vi "sound and graphics.vi"() -> ()   [LabVIEW 2018]
panel:
  out "new picture":picture
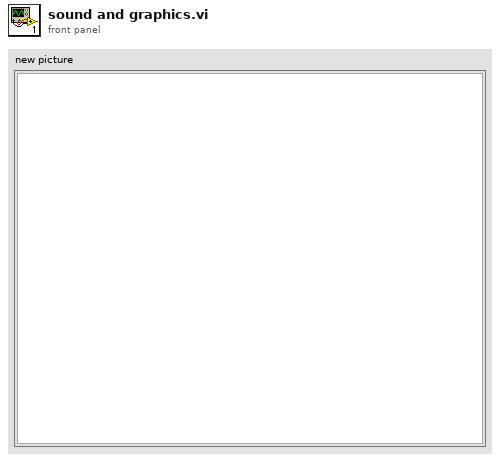
[diagram p1: front panel]
types:
  T1 = typedef "imagedata.ctl" = cluster{"image type":i32, "image depth":i32, "image":u8[], "mask":u8[], "colors":u32[], "Rectangle":cluster{"left":i16, "top":i16, "right":i16, "bottom":i16}}
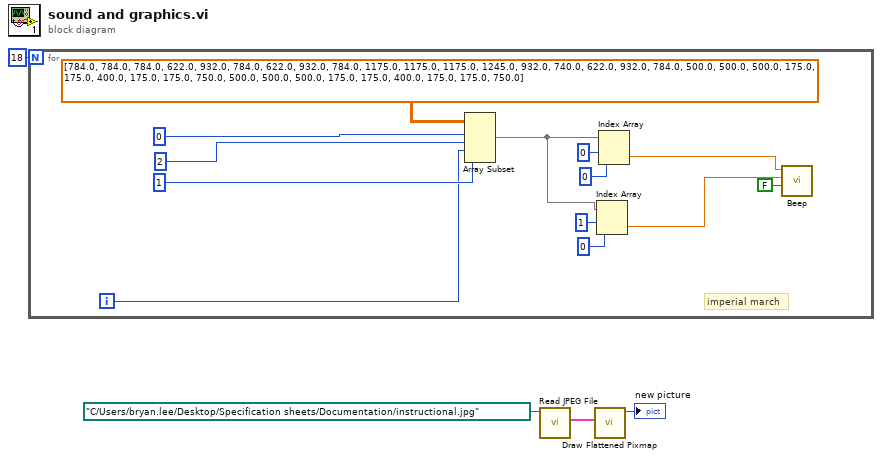
[diagram p0: block diagram]
diagram:
  n1 = for {
    N: 18 -> [_]
    i -> [w9]
    # "imperial march"
    n2 = Array Subset(array=dbl[][] [[784.0, 784.0, 784.0, 622.0, 932.0, 784.0, 622.0, 932.0, 784.0, 1175.0, 1175.0, 1175.0, 1245.0, 932.0, 740.0, 622.0, 932.0, 784.0], [500.0, 500.0, 500.0, 175.0, 175.0, 400.0, 175.0, 175.0, 750.0, 500.0, 500.0, 500.0, 175.0, 175.0, 400.0, 175.0, 175.0, 750.0]] ("Array"), index (row)=0 ("index"), length (row)=2 ("length"), index (col)=w9, length (col)=1 ("length")) -> (w10:dbl[][])
    n3 = Index Array(array=w10, index (row)=1, index (col)=0 ("disabled index (col)")) -> (element=w5:dbl)
    n4 = Index Array(array=w10, index (row)=0, index (col)=0 ("disabled index (col)")) -> (element=w6:dbl)
    n5 = call <vilib>:"Beep.vi"("use system alert? (T)"=FALSE, "duration (msec)"=w5, "frequency (Hz)"=w6) -> ()  [unwired: 9 in]
  }
  n6 = call <vilib>:"Read JPEG File.vi"("path to JPEG file"=path "C:/Users/bryan.lee/Desktop/Specification sheets/Documentation/instructional.jpg") -> ("image data"=w3:T1)  [unwired: 8 in, 2 out]
  n7 = call <vilib>:"Draw Flattened Pixmap.vi"("image data"=w3) -> ("new picture"=→"new picture":picture)  [unwired: 8 in]
